vi "FP_InitCapture.vi"(7 "ComponentType":u32=12, 8 "error out 2":errorcluster, 11 "connection ID":refnum<k5>) -> (0 "error out":errorcluster, 1 "Data":string, 3 "connection ID out":refnum<k5>, 4 "Data 3":string)   [LabVIEW 2010]
panel:
  out "Data 5":string
  out "Data 4":string
  out "Data 2":string
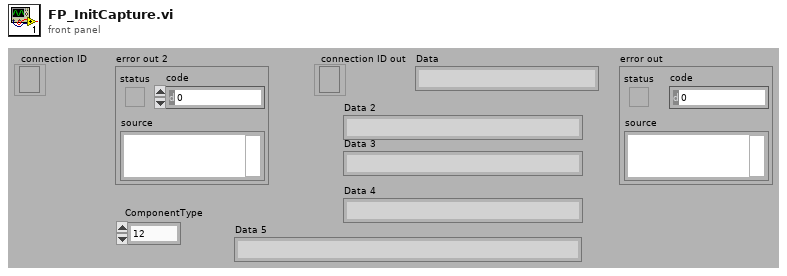
[diagram p1: front panel]
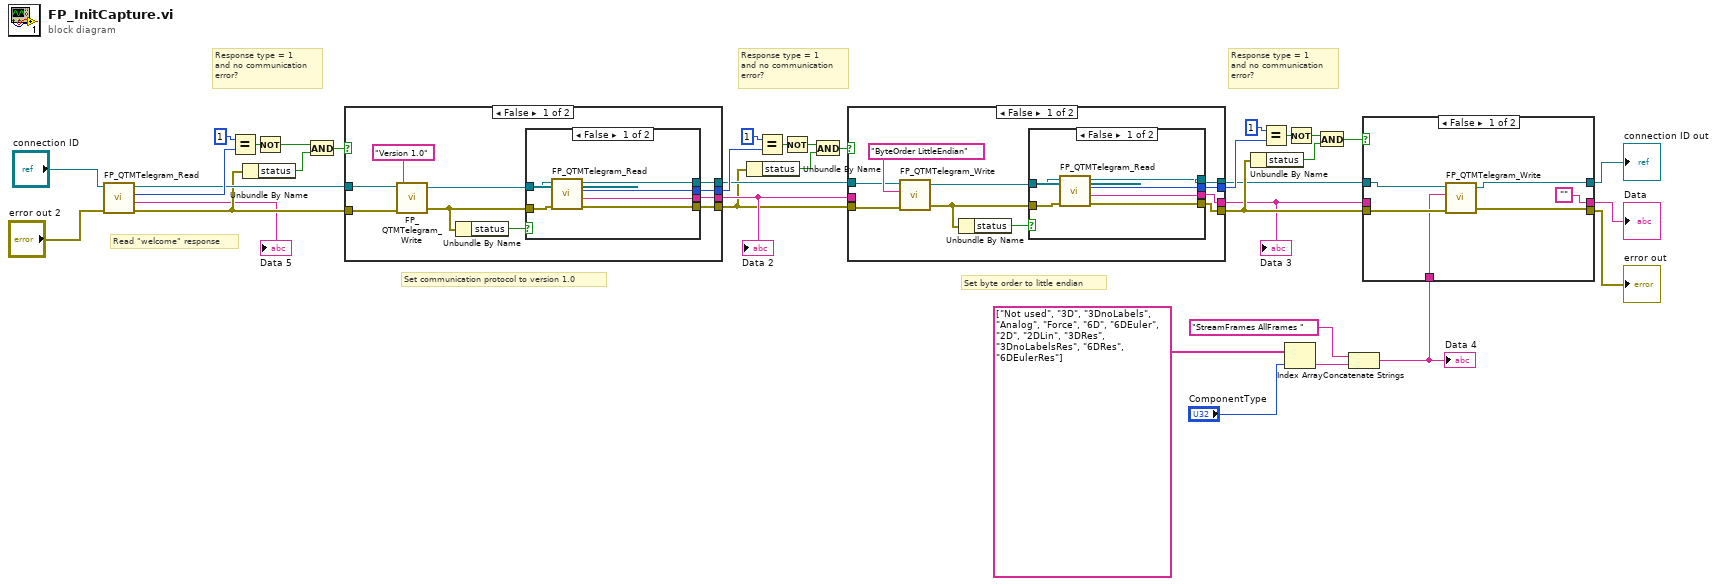
[diagram p0: block diagram]
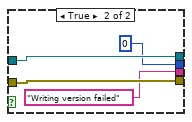
[diagram p3: hidden frame]
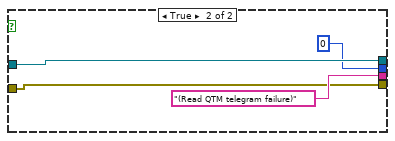
[diagram p4: hidden frame]
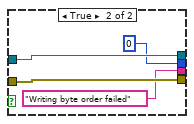
[diagram p5: hidden frame]
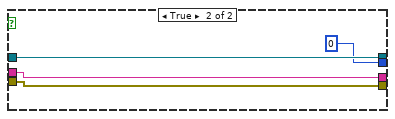
[diagram p6: hidden frame]
diagram:
  # "Response type = 1\nand no communication\nerror?"
  # "Set byte order to little endian"
  # "Response type = 1\nand no communication\nerror?"
  # "Response type = 1\nand no communication\nerror?"
  # "Set communication protocol to version 1.0"
  # "Read \"welcome\" response"
  n1 = call "FP_QTMTelegram_Read.vi"("error in (no error)"="error out 2", "connection ID in"="connection ID") -> ("error out"=w17:errorcluster, "Data"=→"Data 5":string, "Response type"=w19:i32, "connection ID out"=w18:refnum<k5>)  [unwired: 1 in, 5 out]
  n2 = Equal?(x=1, y=w19) -> (x = y?=w20:bool)
  n3 = Unbundle By Name(w17) -> ("status"=w22:bool)
  n4 = Not(x=w20) -> (.not. x?=w21:bool)
  n5 = And(x=w21, y=w22) -> (x .and. y?=w26:bool)
  n6 = case shown="False" w26 {
    tunnel: w17 -> [w47 w59]
    tunnel: w18 -> [w46 w60]
    tunnel: [w41 w59] -> w23
    tunnel: [w40 w60] -> w24
    tunnel: [w39 "(Read QTM telegram failure)" ("Data")] -> w25
    tunnel: [w38 0 ("Response type")] -> w30
    frame False {
      n7 = call "FP_QTMTelegram_Write.vi"("error in (no error)"=w47, "String to send"="Version 1.0" ("data in"), "connection ID"=w46) -> ("error out"=w43:errorcluster, "connection ID out"=w42:refnum<k5>)  [unwired: 1 in, 1 out]
      n8 = Unbundle By Name(w43) -> ("status"=w45:bool)
      n9 = case shown="False" w45 {
        tunnel: w43 -> [w49 w56]
        tunnel: w42 -> [w53 w57]
        tunnel: [w52 w57] -> w40
        tunnel: [w51 w56] -> w41
        tunnel: [w50 "Writing version failed" ("Data")] -> w39
        tunnel: [w48 0 ("Response type")] -> w38
        frame False {
          n10 = call "FP_QTMTelegram_Read.vi"("error in (no error)"=w49, "connection ID in"=w53) -> ("error out"=w51:errorcluster, "Data"=w50:string, "Response type"=w48:i32, "connection ID out"=w52:refnum<k5>)  [unwired: 1 in, 5 out]
        }
        frame True {
        }
      }
    }
    frame True {
    }
  }
  "Data 2" <- w25
  n11 = Unbundle By Name(w23) -> ("status"=w31:bool)
  n12 = Equal?(x=1, y=w30) -> (x = y?=w28:bool)
  n13 = Not(x=w28) -> (.not. x?=w27:bool)
  n14 = And(x=w27, y=w31) -> (x .and. y?=w32:bool)
  n15 = case shown="False" w32 {
    tunnel: w23 -> [w67 w83]
    tunnel: w24 -> [w66 w85]
    tunnel: w25 -> [_ w84]
    tunnel: [w65 w84] -> w11
    tunnel: [w64 w85] -> w10
    tunnel: [w63 w83] -> w12
    tunnel: [w62 0 ("Response type")] -> w37
    frame False {
      n16 = call "FP_QTMTelegram_Write.vi"("error in (no error)"=w67, "String to send"="ByteOrder LittleEndian" ("data in"), "connection ID"=w66) -> ("error out"=w70:errorcluster, "connection ID out"=w71:refnum<k5>)  [unwired: 1 in, 1 out]
      n17 = Unbundle By Name(w70) -> ("status"=w68:bool)
      n18 = case shown="False" w68 {
        tunnel: w70 -> [w76 w80]
        tunnel: w71 -> [w77 w81]
        tunnel: [w75 w81] -> w64
        tunnel: [w74 w80] -> w63
        tunnel: [w73 "Writing byte order failed" ("Data")] -> w65
        tunnel: [w72 0 ("Response type")] -> w62
        frame False {
          n19 = call "FP_QTMTelegram_Read.vi"("error in (no error)"=w76, "connection ID in"=w77) -> ("error out"=w74:errorcluster, "Data"=w73:string, "Response type"=w72:i32, "connection ID out"=w75:refnum<k5>)  [unwired: 1 in, 5 out]
        }
        frame True {
        }
      }
    }
    frame True {
    }
  }
  "Data 3" <- w11
  n20 = Unbundle By Name(w12) -> ("status"=w33:bool)
  n21 = Equal?(x=1, y=w37) -> (x = y?=w35:bool)
  n22 = Index Array(array=string[] ["Not used", "3D", "3DnoLabels", "Analog", "Force", "6D", "6DEuler", "2D", "2DLin", "3DRes", "3DnoLabelsRes", "6DRes", "6DEulerRes"], index="ComponentType") -> (element=w2:string)
  n23 = Not(x=w35) -> (.not. x?=w36:bool)
  n24 = And(x=w36, y=w33) -> (x .and. y?=w13:bool)
  n25 = Concatenate Strings("StreamFrames AllFrames " ("data in"), w2) -> (w1:string)
  "Data 4" <- w1
  n26 = case shown="False" w13 {
    tunnel: w12 -> [w91 w93]
    tunnel: w11 -> [_ w94]
    tunnel: ["" w94] -> w8
    tunnel: [w90 w93] -> w7
    tunnel: w10 -> [w88 w92]
    tunnel: [w87 w92] -> w9
    tunnel: w1 -> [w86 _]
    frame False {
      n27 = call "FP_QTMTelegram_Write.vi"("error in (no error)"=w91, "String to send"=w86, "connection ID"=w88) -> ("error out"=w90:errorcluster, "connection ID out"=w87:refnum<k5>)  [unwired: 1 in, 1 out]
    }
    frame True {
    }
  }
  "error out" <- w7
  "Data" <- w8
  "connection ID out" <- w9
